vi "CPP_Aeroprobe_dT-Unified.vi"() -> (5 "Plug in titles":string[](array[string]), 7 "Plug in values":string[](array[string]))   [LabVIEW 2014]
uses:
  Plug in sub vis/CPP_Aeroprobe/SanityCluster.ctl
  <vilib>/Analysis/baseanly.llb/Mean (DBL).vi
  Globals/Meas_global.vi
  Globals/Trav_pos_global.vi
  <vilib>/Utility/file.llb/Write To Spreadsheet File (DBL).vi
  <vilib>/Analysis/NI_AALBase.lvlib
panel:
  in  "SaveTimeSeries?":bool
  in  "Mode":enum32{"Measure", "Take Zeroes"}(radio)
  in  "RunManually?":bool
  in  "MeanOrFull":bool
  in  "Graphs":bool
  in  "Downsampler":i32=80
  in  "Calibration Folder Path":path=path "M:/Preferences/Rig_Setups/All_Rigs/Calibrations/5HoleProbeRegrid"
  in  "Correction File Path":path=path "M:/Preferences/Rig_Setups/All_Rigs/TubingCompensation/5HPTubingCorrection12066.xls"
  # "!! 5-hole 1-5 must be connected to Channels 1-5 !!"
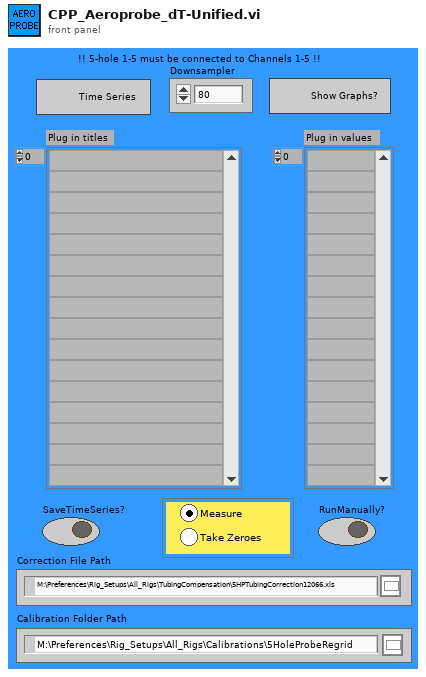
[diagram p1: front panel]
types:
  T1 = enum16{"Save no data", "Save data in new files", "Save data in existing files"}
  T2 = typedef "SanityCluster.ctl" = cluster{"PressureErrors":bool[][], "Plug in titles":string[]}
  T3 = typedef "Post_Process.ctl" = enum16{"Take New Data", "Post Process Raw Data File"}
  T4 = typedef "Traverse_cluster.ctl" = cluster{"Start X":sgl, "Start Y":sgl, "Start Z":sgl, "End X":sgl, "End Y":sgl, "End Z":sgl, "No. of pts.":i32, "Spacing":T5, "Filename":path, "Tunnel Speed":dbl, "Averaging time (min)":dbl, "Extra Commands":string, "Specific Arguments":string, "Emission Rate (l/min)":dbl, "Trace Gas Concentration (%)":dbl, "Density Ratio":string, "Comments":string, "Row No":i32, "Row Type Selector":T6, "Completion time":string, "Row Duration (mins)":dbl, "No. of Valid pts.":i32, "Meas Setup File":string}
  T5 = typedef "Spacing.ctl" = enum16{"Linear", "Log", "Gauss", "Specified", "N/A"}
  T6 = typedef "Multi_run_mode.ctl" = enum16{"Move Traverse Only", "Set Tunnel Speed Only", "Set Source Only", "Set Measurement Conditions", "Single Measurement", "Vertical Profile", "Lateral Profile", "Longitudinal Profile", "Explore Volume", "Multi-Axis Profile", "Auto Calibrate", "Meas Fast FID Bkgnd", "Check Beam Power", "Scanning Valve Measurement", "Run VI Named:", "Set ADAM Ch", "Wait (minutes)", "Send Message", "Synchronize With:", "Fall Back to this Row", "Turn Off Row Repeating", "Blank Row", "Traverse 3D Volume"}
  T7 = typedef "Analysis_info_cluster.ctl" = cluster{"Colour":u32, "Inst type":T8, "Inst name":string, "Symbol":string, "Code name":string, "Extra Info":string, "Inst Array":T9, "Extra Titles":string[], "Extra Values":string[], "U":dbl, "u^2":dbl, "u^3":dbl, "u^4":dbl, "Skew_u":dbl, "Kurt_u":dbl, "Sd Error in Mean":dbl, "% u'/U":dbl, "X":dbl, "Y":dbl, "Z":dbl, "Timescale integral to 25%":dbl, "Sd Error in Variance":dbl, "Calib File":path, "Calib Constants":dbl[], "Output Position":bool, "Full Stats":bool, "Av Sampling Rate":dbl, "Av No of Samples":dbl, "Total Meas Time (s)":dbl, "ADAM Ch Name":string}
  T8 = typedef "Inst_type.ctl" = enum16{"Propeller anemometer", "Raw voltage", "Pressure Transducer", "Pitot-static tube", "Preston tube", "Hot wire", "Cross wire 1", "Cross wire 2", "Generic Linear", "Generic Polynomial", "Generic BackPoly", "Fast FID", "Thermocouple", "Cold wire", "Pulsed Wire", "LDA Vel", "LDA Tran time", "LDA Arr time", "Microphone"}
  T9 = typedef "Instrument_Array.ctl" = enum16{"PWA", "LDA", "Analogue"}
  T10 = cluster{"Analysis Info cluster[0]":T7, "Analysis Info cluster[1]":T7, "Analysis Info cluster[2]":T7, "Analysis Info cluster[3]":T7, "Analysis Info cluster[4]":T7, "Analysis Info cluster[5]":T7, "Analysis Info cluster[6]":T7}
  T11 = typedef "Time_Trace_Cluster.ctl" = cluster{"Weighting":dbl[], "Time (s)":dbl[], "Voltage":dbl[], "Eng Values":dbl[]}
  T12 = typedef "GoodArray.ctl" = bool[]
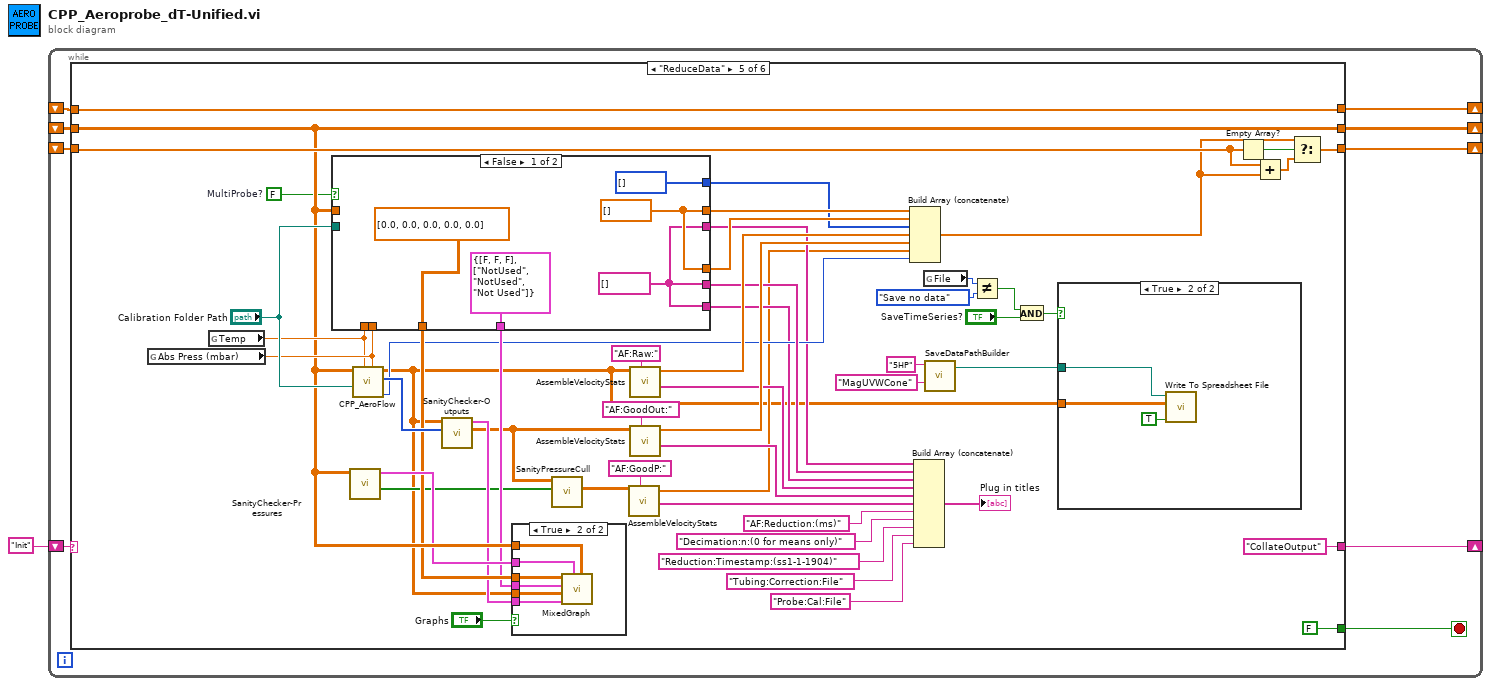
[diagram p0: block diagram]
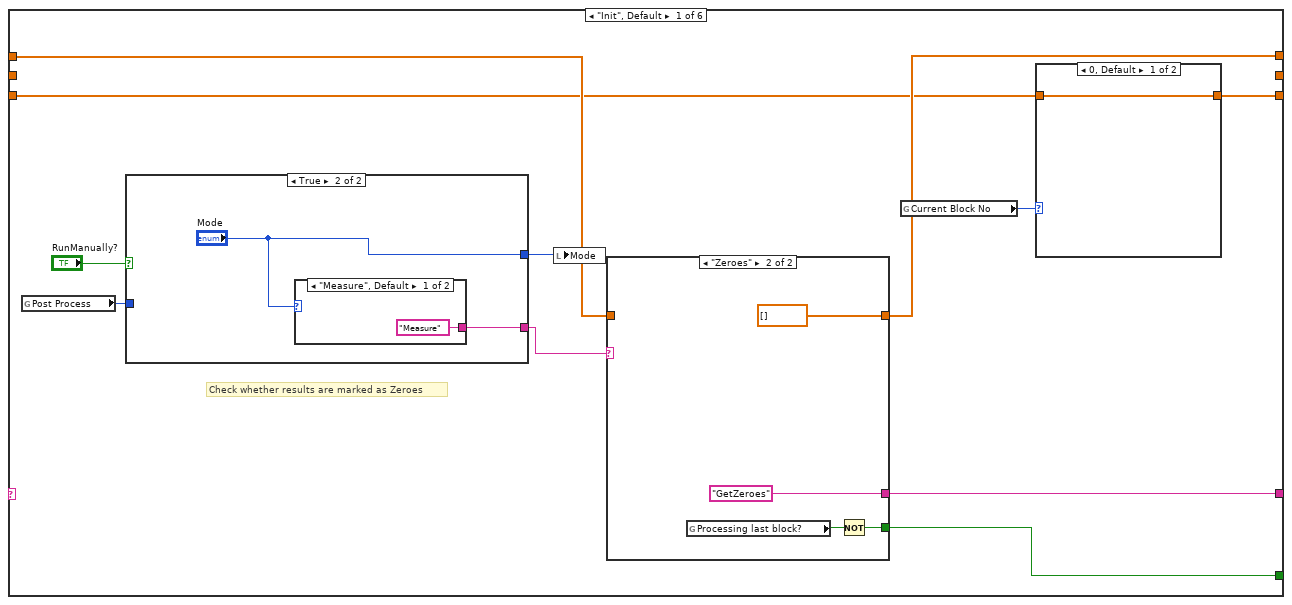
[diagram p2: hidden frame]
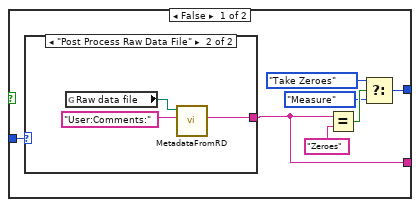
[diagram p3: hidden frame]
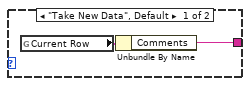
[diagram p4: hidden frame]
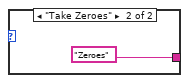
[diagram p5: hidden frame]
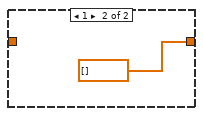
[diagram p6: hidden frame]
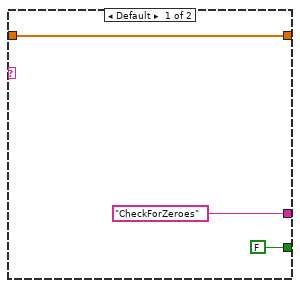
[diagram p7: hidden frame]
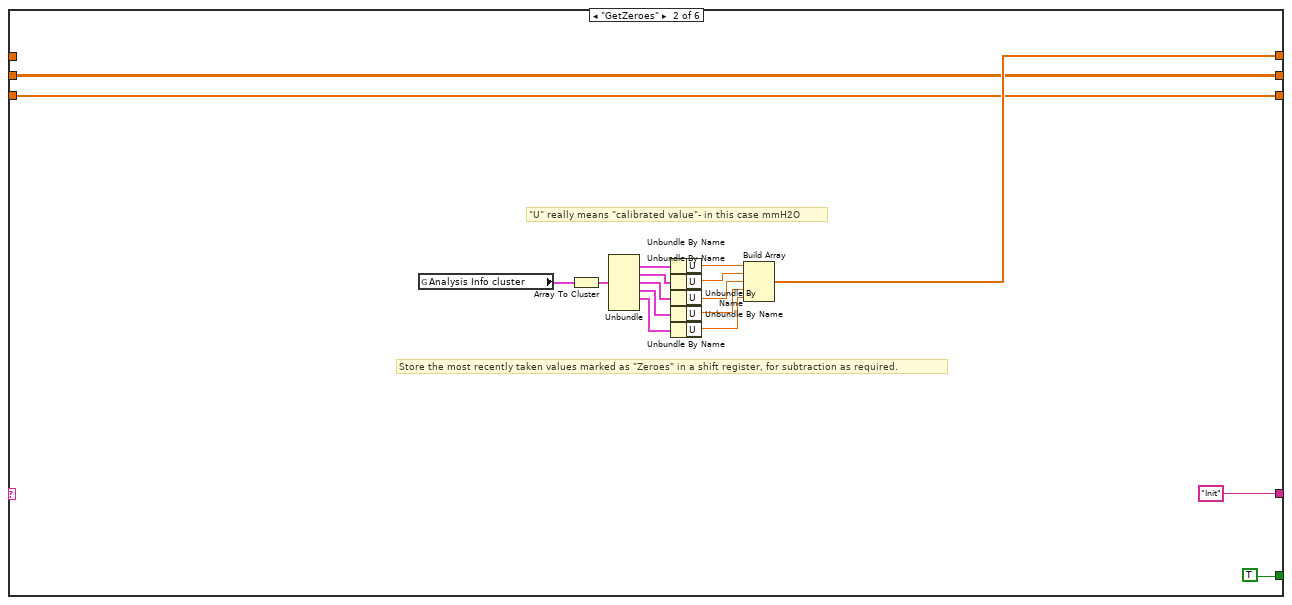
[diagram p8: hidden frame]
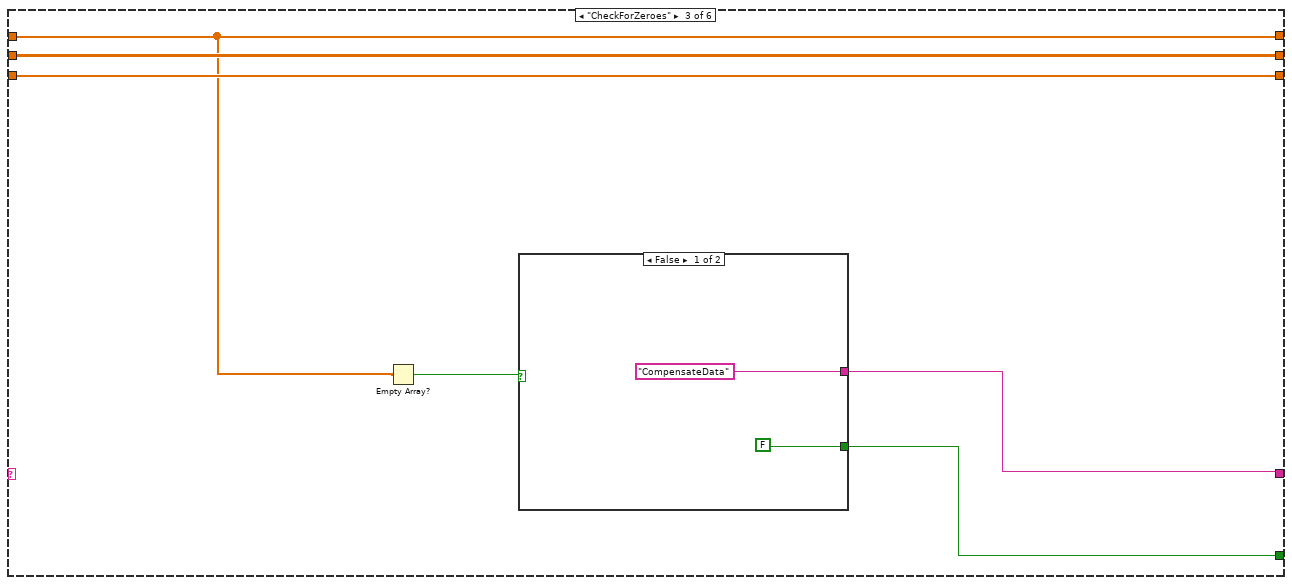
[diagram p9: hidden frame]
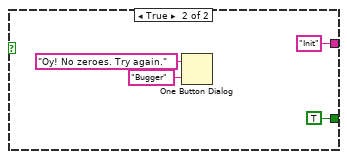
[diagram p10: hidden frame]
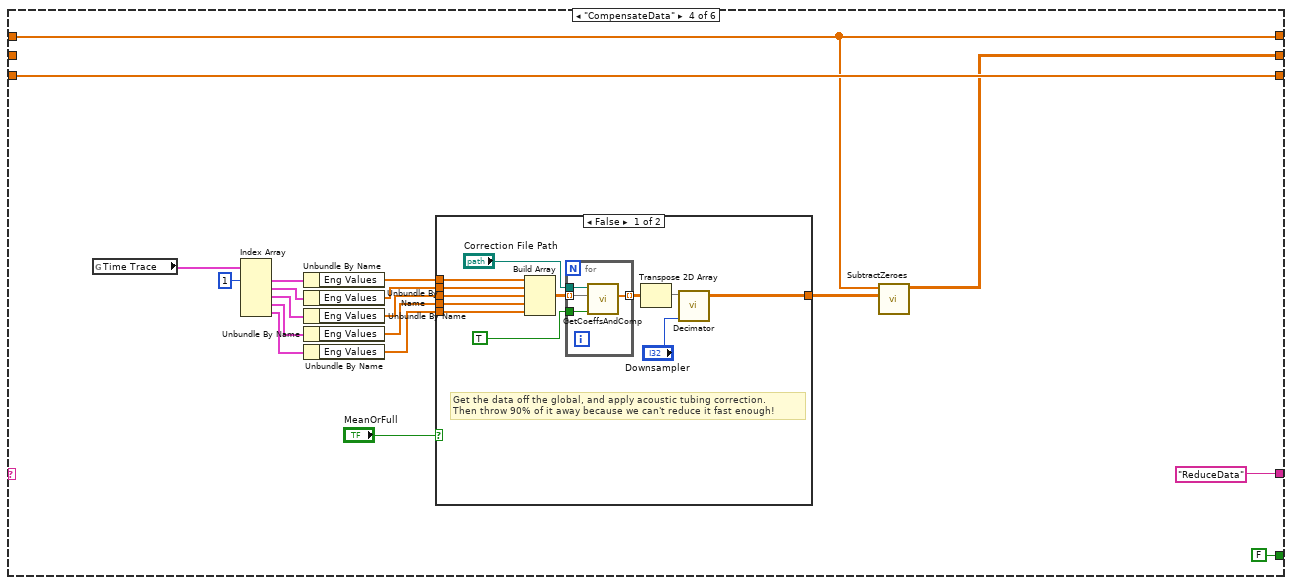
[diagram p11: hidden frame]
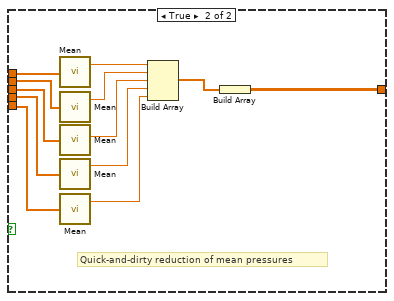
[diagram p12: hidden frame]
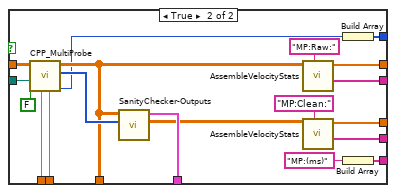
[diagram p14: hidden frame]
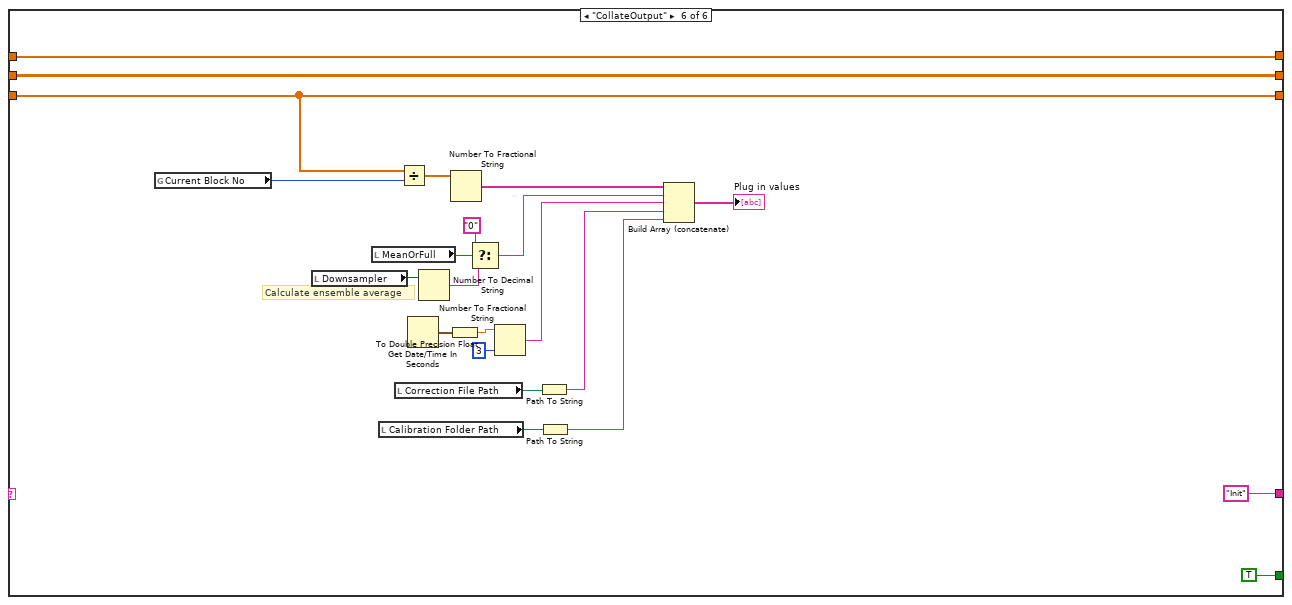
[diagram p16: hidden frame]
diagram:
  n1 = while {
    shift-right: [w9] -> _
    shift-left: "Init" -> [w10]
    shift-right: [w8] -> _
    shift-left: _ -> [w7]
    shift-right: [w6] -> _
    shift-left: _ -> [w5]
    shift-right: [w3] -> _
    shift-left: _ -> [w2]
    stop <- w4 stop-if-true
    n2 = case shown="\"ReduceData\"" w10 {
      tunnel: [w21 "Init" w68 "ReduceData" "CollateOutput" "Init"] -> w9
      tunnel: [w18 w50 w65 w80 w174 w230] -> w8
      tunnel: w7 -> [w19 _ w65 w80 w174 w230]
      tunnel: [w17 w48 w69 w94 w169 w224] -> w6
      tunnel: w5 -> [w16 w48 w69 w94 w172 w224]
      tunnel: [w20 TRUE w67 FALSE FALSE TRUE] -> w4
      tunnel: [_ w47 w66 w77 w161 w226] -> w3
      tunnel: w2 -> [_ w47 w66 _ w161 w226]
      frame "Init", Default {
        # "Check whether results are marked as Zeroes"
        n3 = global read "Meas_global.vi" "Post Process"() -> (w12:T3)
        n4 = case shown="True" "RunManually?" {
          tunnel: [w28 "Mode"] -> w13
          tunnel: w12 -> [w23 _]
          tunnel: [w22 w34] -> w11
          frame False {
            n5 = case shown="\"Post Process Raw Data File\"" w23 {
              tunnel: [w29 w31] -> w22
              frame "Take New Data", Default {
                n6 = global read "Trav_pos_global.vi" "Current Row"() -> (w30:T4)
                n7 = Unbundle By Name(w30) -> ("Comments"=w29:string)
              }
              frame "Post Process Raw Data File" {
                n8 = global read "Meas_global.vi" "Raw data file"() -> (w33:path)
                n9 = call "MetadataFromRD.vi"("ChannelName"="User:Comments:", "Raw data file"=w33) -> ("ValueString"=w31:string)  [unwired: 8 in, 1 out]
              }
            }
            n10 = Equal?(x=w22, y="Zeroes") -> (x = y?=w26:bool)
            n11 = Select(t=enum32{"Measure", "Take Zeroes"}."Take Zeroes" ("Mode"), s=w26, f=enum32{"Measure", "Take Zeroes"}."Measure" ("Mode")) -> (s? t:f=w28:enum32{"Measure", "Take Zeroes"})
          }
          frame True {
            n12 = case shown="\"Measure\", Default" "Mode" {
              tunnel: ["Measure" ("y") "Zeroes" ("y")] -> w34
              frame "Measure", Default {
              }
              frame "Take Zeroes" {
              }
            }
          }
        }
        n13 = local write "Mode"(w13) -> ()
        n14 = case shown="\"Zeroes\"" w11 {
          tunnel: ["CheckForZeroes" "GetZeroes"] -> w21
          tunnel: [FALSE w45] -> w20
          tunnel: w19 -> [w40 _]
          tunnel: [w40 dbl[] [] ("t")] -> w18
          frame Default {
          }
          frame "Zeroes" {
            n15 = global read "Meas_global.vi" "Processing last block?"() -> (w44:bool)
            n16 = Not(x=w44) -> (.not. x?=w45:bool)
          }
        }
        n17 = global read "Meas_global.vi" "Current Block No"() -> (w15:i32)
        n18 = case shown="0, Default" w15 {
          tunnel: [w38 dbl[] [] ("t")] -> w17
          tunnel: w16 -> [w38 _]
          frame 0, Default {
          }
          frame 1 {
          }
        }
      }
      frame "GetZeroes" {
        # "Store the most recently taken values marked as \"Zeroes\" in a shift register, for subtraction as required."
        # "\"U\" really means \"calibrated value\"- in this case mmH2O"
        n19 = global read "Meas_global.vi" "Analysis Info cluster"() -> (w52:T7[])
        n20 = Array To Cluster(array=w52) -> (cluster=w58:T10)
        n21 = Unbundle(w58) -> ("Analysis Info cluster[1]"=w59:T7, "Analysis Info cluster[2]"=w60:T7, "Analysis Info cluster[3]"=w61:T7, "Analysis Info cluster[4]"=w62:T7, "Analysis Info cluster[5]"=w63:T7)  [unwired: 2 out]
        n22 = Unbundle By Name(w59) -> ("U"=w57:dbl)
        n23 = Unbundle By Name(w60) -> ("U"=w56:dbl)
        n24 = Unbundle By Name(w61) -> ("U"=w55:dbl)
        n25 = Unbundle By Name(w62) -> ("U"=w54:dbl)
        n26 = Unbundle By Name(w63) -> ("U"=w53:dbl)
        n27 = Build Array(w57, w56, w55, w54, w53) -> (w50:dbl[])
      }
      frame "CheckForZeroes" {
        n28 = Empty Array?(array=w65) -> (empty?=w64:bool)
        n29 = case shown="False" w64 {
          tunnel: ["CompensateData" "Init"] -> w68
          tunnel: [FALSE TRUE] -> w67
          frame False {
          }
          frame True {
            n30 = One Button Dialog(message="Oy! No zeroes. Try again.", button name ("OK")="Bugger") -> ()  [unwired: 1 out]
          }
        }
      }
      frame "CompensateData" {
        n31 = global read "Meas_global.vi" "Time Trace"() -> (w84:T11[])
        n32 = Index Array(array=w84, index #1=1 ("index")) -> (element #1=w83:T11, element #2=w92:T11, element #3=w91:T11, element #4=w90:T11, element #5=w89:T11)  [unwired: 4 in]
        n33 = Unbundle By Name(w83) -> ("Eng Values"=w82:dbl[])
        n34 = Unbundle By Name(w92) -> ("Eng Values"=w88:dbl[])
        n35 = Unbundle By Name(w91) -> ("Eng Values"=w87:dbl[])
        n36 = Unbundle By Name(w90) -> ("Eng Values"=w86:dbl[])
        n37 = Unbundle By Name(w89) -> ("Eng Values"=w85:dbl[])
        n38 = case shown="False" "MeanOrFull" {
          tunnel: w88 -> [w106 w121]
          tunnel: w87 -> [w105 w120]
          tunnel: w86 -> [w104 w119]
          tunnel: w85 -> [w103 w118]
          tunnel: w82 -> [w102 w122]
          tunnel: [w95 w111] -> w81
          frame False {
            # "Get the data off the global, and apply acoustic tubing correction. \nThen throw 90% of it away because we can't reduce it fast enough!"
            n39 = Build Array(w102, w106, w105, w104, w103) -> (w101:dbl[][])
            n40 = for {
              tunnel: w101 -> [w110] mode=indexing
              tunnel: [w109] -> w98 mode=indexing
              tunnel: TRUE ("Apply Phase Correction?") -> [w108]
              tunnel: "Correction File Path" -> [w107]
              n41 = call "GetCoeffsAndComp.vi"("Apply Phase Correction?"=w108, "mutedData"=w110, "TubingCorrectionFile"=w107) -> ("boostedData"=w109:dbl[])  [unwired: 8 in]
            }
            n42 = Transpose 2D Array(2D array=w98) -> (transposed array=w97:dbl[][])
            n43 = call "Decimator.vi"("Decimator"="Downsampler", "Array In"=w97) -> ("DecimatedArrayOut"=w95:dbl[][])  [unwired: 9 in]
          }
          frame True {
            # "Quick-and-dirty reduction of mean pressures"
            n44 = call-poly <vilib>:"Mean.vi"("X"=w122) -> ("mean"=w117:dbl)  [unwired: 1 out]
            n45 = call-poly <vilib>:"Mean.vi"("X"=w121) -> ("mean"=w116:dbl)  [unwired: 1 out]
            n46 = call-poly <vilib>:"Mean.vi"("X"=w120) -> ("mean"=w115:dbl)  [unwired: 1 out]
            n47 = call-poly <vilib>:"Mean.vi"("X"=w119) -> ("mean"=w114:dbl)  [unwired: 1 out]
            n48 = call-poly <vilib>:"Mean.vi"("X"=w118) -> ("mean"=w113:dbl)  [unwired: 1 out]
            n49 = Build Array(w117, w116, w115, w114, w113) -> (w112:dbl[])
            n50 = Build Array(w112) -> (w111:dbl[][])
          }
        }
        n51 = call "SubtractZeroes.vi"("RawPressure"=w81, "Zeroes"=w80) -> ("ZeroedPressure"=w77:dbl[][])  [unwired: 9 in]
      }
      frame "ReduceData" {
        w143 = FALSE  # MultiProbe?
        n52 = global read "Meas_global.vi" "Abs Press (mbar)"() -> (w166:dbl)
        n53 = global read "Meas_global.vi" "Temp"() -> (w165:dbl)
        n54 = case shown="False" w143 {
          tunnel: [w183 w202] -> w168
          tunnel: "Calibration Folder Path" -> [_ w201]
          tunnel: w166 -> [_ w200]
          tunnel: w165 -> [_ w199]
          tunnel: w161 -> [_ w195]
          tunnel: [dbl[][] [[0.0, 0.0, 0.0, 0.0, 0.0]] ("RawVmagUVWCone") w194] -> w159
          tunnel: [T2 {"PressureErrors"=[[FALSE, FALSE, FALSE]], "Plug in titles"=["NotUsed", "NotUsed", "Not Used"]} ("OutputErrors") w193] -> w158
          tunnel: [w183 w190] -> w154
          tunnel: [w182 w189] -> w151
          tunnel: [u32[] [] w185] -> w146
          tunnel: [w182 w184] -> w145
          tunnel: [w182 w186] -> w144
          frame False {
            w182 = string[] [] ("Plug in titles")
            w183 = dbl[] [] ("StatsArray")
          }
          frame True {
            n55 = call "CPP_MultiProbe.vi"("Pressure (mBar)"=w200, "Temperature (C)"=w199, "Old5HoleProbe?"=FALSE, "Calibration Folder Path"=w201, "ZeroedPressures (mmH2O)"=w195) -> ("Time (ms)"=w188:u32, "ReductionCode"=w196:i32[], "RawVmagUVWCone"=w194:dbl[][])  [unwired: 1 in, 1 out]
            n56 = call "SanityChecker-Outputs.vi"("ReductionCode"=w196, "RawVmagUVWCone"=w194) -> ("SanitisedVmagUVWCone"=w192:dbl[][], "OutputErrors"=w193:T2)  [unwired: 7 in, 1 out]
            n57 = call "AssembleVelocityStats.vi"("TitlePrefix"="MP:Raw:", "VmagUVWCone"=w194) -> ("Plug in titles"=w186:string[], "StatsArray"=w202:dbl[])  [unwired: 8 in]
            n58 = call "AssembleVelocityStats.vi"("TitlePrefix"="MP:Clean:", "VmagUVWCone"=w192) -> ("Plug in titles"=w189:string[], "StatsArray"=w190:dbl[])  [unwired: 8 in]
            n59 = Build Array(w188) -> (w185:u32[])
            n60 = Build Array("MP:(ms)") -> (w184:string[])
          }
        }
        n61 = call "SanityChecker-Pressures.vi"("ZeroedPressures"=w161) -> ("GoodPressures"=w139:T12, "Sanity"=w160:T2)  [unwired: 9 in]
        n62 = call "CPP_AeroFlow.vi"("Pressure (mBar)"=w166, "Temperature (C)"=w165, "Calibration Folder Path"="Calibration Folder Path", "ZeroedPressures (mmH2O)"=w161) -> ("Time(ms)"=w147:u32, "ReductionCode"=w163:i32[], "RawVmagUVWCone"=w130:dbl[][])  [unwired: 2 in, 1 out]
        n63 = call "SanityChecker-Outputs.vi"("ReductionCode"=w163, "RawVmagUVWCone"=w130) -> ("SanitisedVmagUVWCone"=w140:dbl[][], "OutputErrors"=w157:T2)  [unwired: 7 in, 1 out]
        n64 = case shown="True" "Graphs" {
          tunnel: w161 -> [_ w208]
          tunnel: w160 -> [_ w207]
          tunnel: w159 -> [_ w206]
          tunnel: w158 -> [_ w205]
          tunnel: w130 -> [_ w204]
          tunnel: w157 -> [_ w203]
          frame False {
          }
          frame True {
            n65 = call "MixedGraph.vi"("ZeroedPressure"=w208, "PressureSanity"=w207, "OutputErrors2"=w203, "RawVmagUVWCone2"=w204, "OutputErrors1"=w205, "RawVmagUVWCone1"=w206) -> ()  [unwired: 6 in]
          }
        }
        n66 = call "SanityPressureCull.vi"("GoodPressures"=w139, "VmagUVWCone"=w140) -> ("SanitisedVmagUVWCone"=w141:dbl[][])  [unwired: 9 in]
        n67 = call "AssembleVelocityStats.vi"("TitlePrefix"="AF:GoodP:", "VmagUVWCone"=w141) -> ("Plug in titles"=w138:string[], "StatsArray"=w136:dbl[])  [unwired: 8 in]
        n68 = call "AssembleVelocityStats.vi"("TitlePrefix"="AF:Raw:", "VmagUVWCone"=w130) -> ("Plug in titles"=w150:string[], "StatsArray"=w153:dbl[])  [unwired: 8 in]
        n69 = call "AssembleVelocityStats.vi"("TitlePrefix"="AF:GoodOut:", "VmagUVWCone"=w140) -> ("Plug in titles"=w149:string[], "StatsArray"=w152:dbl[])  [unwired: 8 in]
        n70 = Build Array (concatenate)(w168, w154, w146, w153, w152, w136, w147) -> (w155:dbl[])
        n71 = Build Array (concatenate)(w144, w151, w145, w150, w149, w138, "AF:Reduction:(ms)", "Decimation:n:(0 for means only)" ("element"), "Reduction:Timestamp:(ss1-1-1904)" ("element"), "Tubing:Correction:File" ("element"), "Probe:Cal:File" ("element")) -> (→"Plug in titles":string[])
        n72 = global read "Meas_global.vi" "File"() -> (w126:T1)
        n73 = call "SaveDataPathBuilder.vi"("DataTypeSuffix"="MagUVWCone", "Inst name"="5HP") -> ("Path name Out"=w129:path)  [unwired: 9 in]
        n74 = Not Equal?(x=w126, y=T1."Save no data" ("File")) -> (x != y?=w123:bool)
        n75 = And(x=w123, y="SaveTimeSeries?") -> (x .and. y?=w124:bool)
        n76 = case shown="True" w124 {
          tunnel: w130 -> [_ w178]
          tunnel: w129 -> [_ w177]
          frame False {
          }
          frame True {
            n77 = call-poly <vilib>:"Write To Spreadsheet File.vi"("append to file? (new file:F)"=TRUE, "2D data"=w178, "file path (dialog if empty)"=w177) -> ()  [unwired: 5 in, 1 out]
          }
        }
        n78 = Empty Array?(array=w172) -> (empty?=w171:bool)
        n79 = Add(x=w172, y=w155) -> (x+y=w170:dbl[])
        n80 = Select(t=w155, s=w171, f=w170) -> (s? t:f=w169:dbl[])
      }
      frame "CollateOutput" {
        # "Calculate ensemble average"
        n81 = global read "Meas_global.vi" "Current Block No"() -> (w227:i32)
        n82 = local read "Downsampler"() -> (w223:i32)
        n83 = local read "MeanOrFull"() -> (w222:bool)
        n84 = local read "Calibration Folder Path"() -> (w211:path)
        n85 = local read "Correction File Path"() -> (w213:path)
        n86 = Divide(x=w224, y=w227) -> (x/y=w225:dbl[])
        n87 = Get Date/Time In Seconds() -> (seconds since 1Jan1904=w219:timestamp)
        n88 = Number To Decimal String(number=w223) -> (decimal integer string=w221:string)  [unwired: 1 in]
        n89 = To Double Precision Float(number=w219) -> (double precision float=w218:dbl)
        n90 = Number To Fractional String(number=w225) -> (F-format string=w214:string[])  [unwired: 3 in]
        n91 = Select(t="0", s=w222, f=w221) -> (s? t:f=w217:string)
        n92 = Number To Fractional String(number=w218, precision (6)=i16 3) -> (F-format string=w216:string)  [unwired: 2 in]
        n93 = Path To String(path=w213) -> (string=w212:string)
        n94 = Path To String(path=w211) -> (string=w210:string)
        n95 = Build Array (concatenate)(w214, w217, w216, w212, w210) -> (→"Plug in values":string[])
      }
    }
  }
